vi "build-diode-scan-pts - v3.vi"(4 "Bar In PD Angle":dbl=180.5 format="%#_13g", 5 "Test Start Delay (s)":dbl=60.0, 6 "Bar In Brewster Angle":dbl=45.0 format="%#_13g", 7 "queue in":T2(array[cluster]), 8 "PD Y":cluster{"stop":dbl, "start":dbl, "step":dbl}, 9 "PD X":cluster{"stop":dbl, "start":dbl, "step":dbl}, 10 "Bar Y":cluster{"stop":dbl, "start":dbl, "step":dbl}, 11 "Bar X":cluster{"stop":dbl, "start":dbl, "step":dbl}) -> (3 "queue out":T2(array[cluster]))   [LabVIEW 2024]
panel:
  in  "next-state-cluster":T1={"next-state"="", "mode-select"=enum."IR", "bypass-confirm"=FALSE, "PDX"=300.0, "PDY"=150.0, "BarX"=300.0, "BarY"=150.0, "BMA"=45.0, "PDA"=85.0, "bar-note"=FALSE}
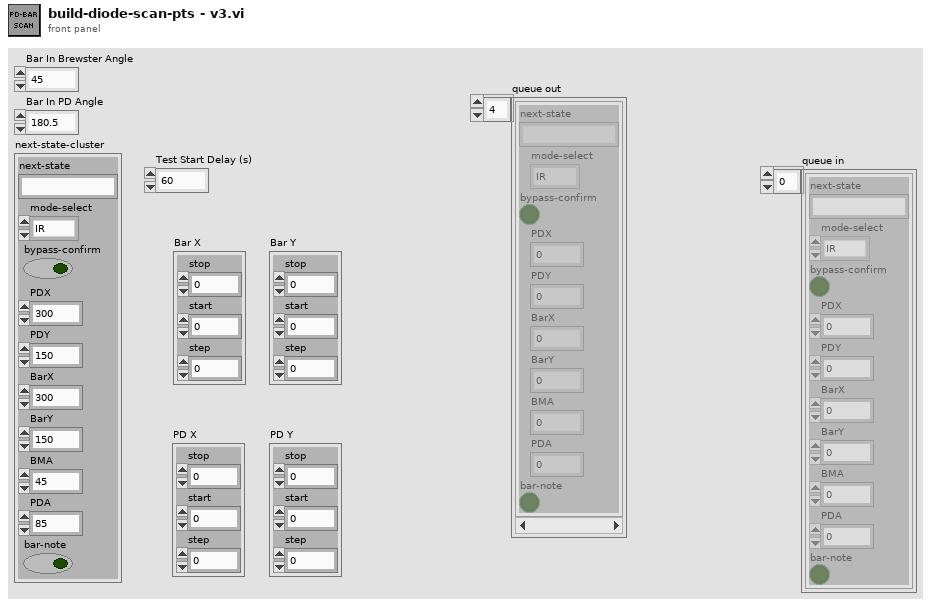
[diagram p1: front panel]
types:
  T1 = cluster{"next-state":string, "mode-select":enum32{"IR", "Pure", "Bulk", "Bar Out", "stored-loc", "custom"}, "bypass-confirm":bool, "PDX":dbl, "PDY":dbl, "BarX":dbl, "BarY":dbl, "BMA":dbl, "PDA":dbl, "bar-note":bool}
  T2 = cluster{"next-state":string, "mode-select":enum32{"IR", "Pure", "Bulk", "Bar Out", "stored-loc", "custom"}, "bypass-confirm":bool, "PDX":dbl, "PDY":dbl, "BarX":dbl, "BarY":dbl, "BMA":dbl, "PDA":dbl, "bar-note":bool}[]
  T3 = enum32{"IR", "Pure", "Bulk", "Bar Out", "stored-loc", "custom"}
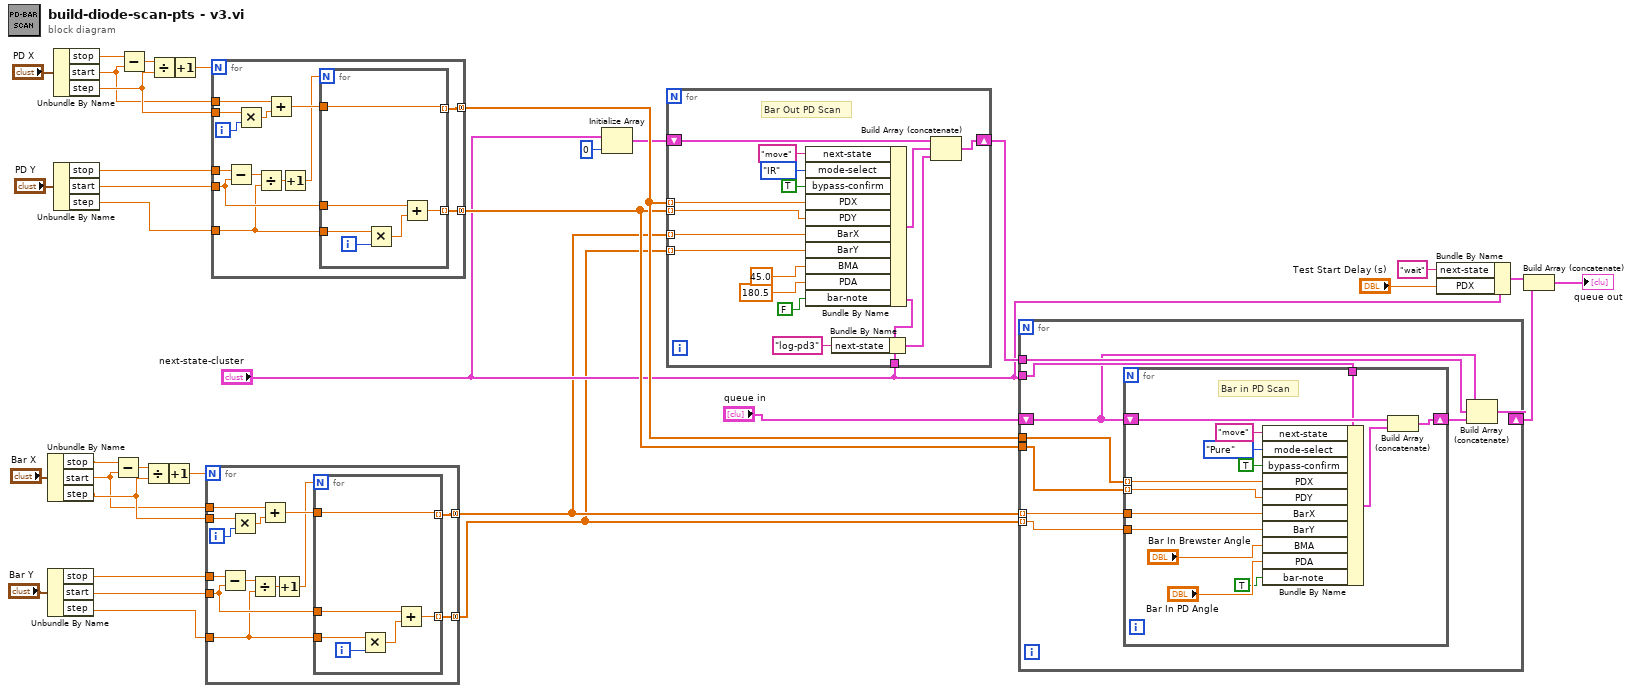
[diagram p0: block diagram]
diagram:
  n1 = Unbundle By Name("Bar X") -> ("stop"=w24:dbl, "start"=w25:dbl, "step"=w26:dbl)
  n2 = Unbundle By Name("Bar Y") -> ("stop"=w27:dbl, "start"=w28:dbl, "step"=w29:dbl)
  n3 = Unbundle By Name("PD X") -> ("stop"=w18:dbl, "start"=w19:dbl, "step"=w20:dbl)
  n4 = Unbundle By Name("PD Y") -> ("stop"=w21:dbl, "start"=w22:dbl, "step"=w23:dbl)
  n5 = Subtract(x=w24, y=w25) -> (x-y=w17:dbl)
  n6 = Subtract(x=w18, y=w19) -> (x-y=w12:dbl)
  n7 = Divide(x=w17, y=w26) -> (x/y=w16:dbl)
  n8 = Divide(x=w12, y=w20) -> (x/y=w13:dbl)
  n9 = Increment(x=w16) -> (x+1=w15:dbl)
  n10 = Increment(x=w13) -> (x+1=w14:dbl)
  n11 = for {
    N: w15 -> [_]
    tunnel: w25 -> [w48]
    tunnel: [w45] -> w2 mode=concatenating
    tunnel: [w44] -> w1 mode=concatenating
    tunnel: w26 -> [w40]
    tunnel: w27 -> [w39]
    tunnel: w28 -> [w38]
    tunnel: w29 -> [w37]
    i -> [w49]
    n12 = Subtract(x=w39, y=w38) -> (x-y=w43:dbl)
    n13 = Multiply(x=w40, y=w49) -> (x*y=w47:dbl)
    n14 = Divide(x=w43, y=w37) -> (x/y=w42:dbl)
    n15 = Add(x=w48, y=w47) -> (x+y=w46:dbl)
    n16 = Increment(x=w42) -> (x+1=w41:dbl)
    n17 = for {
      N: w41 -> [_]
      tunnel: w46 -> [w55]
      tunnel: [w55] -> w45 mode=indexing
      tunnel: [w52] -> w44 mode=indexing
      tunnel: w38 -> [w51]
      tunnel: w37 -> [w50]
      i -> [w53]
      n18 = Multiply(x=w50, y=w53) -> (x*y=w54:dbl)
      n19 = Add(x=w51, y=w54) -> (x+y=w52:dbl)
    }
  }
  n20 = for {
    N: w14 -> [_]
    tunnel: w19 -> [w67]
    tunnel: [w64] -> w9 mode=concatenating
    tunnel: [w63] -> w8 mode=concatenating
    tunnel: w20 -> [w59]
    tunnel: w21 -> [w58]
    tunnel: w22 -> [w57]
    tunnel: w23 -> [w56]
    i -> [w68]
    n21 = Subtract(x=w58, y=w57) -> (x-y=w62:dbl)
    n22 = Multiply(x=w59, y=w68) -> (x*y=w66:dbl)
    n23 = Divide(x=w62, y=w56) -> (x/y=w61:dbl)
    n24 = Add(x=w67, y=w66) -> (x+y=w65:dbl)
    n25 = Increment(x=w61) -> (x+1=w60:dbl)
    n26 = for {
      N: w60 -> [_]
      tunnel: w65 -> [w74]
      tunnel: [w74] -> w64 mode=indexing
      tunnel: [w71] -> w63 mode=indexing
      tunnel: w57 -> [w70]
      tunnel: w56 -> [w69]
      i -> [w72]
      n27 = Multiply(x=w69, y=w72) -> (x*y=w73:dbl)
      n28 = Add(x=w70, y=w73) -> (x+y=w71:dbl)
    }
  }
  n29 = Initialize Array("next-state-cluster", 0 ("dimension size")) -> (w6:T2)
  n30 = for {
    tunnel: w9 -> [w90] mode=indexing
    tunnel: w8 -> [w89] mode=indexing
    shift-right: [w82] -> w11
    shift-left: w6 -> [w84]
    tunnel: "next-state-cluster" -> [w78]
    tunnel: w2 -> [w76] mode=indexing
    tunnel: w1 -> [w75] mode=indexing
    # "Bar Out PD Scan"
    n31 = Bundle By Name(cluster=w78, "next-state"="move", "mode-select"=T3."IR", "bypass-confirm"=TRUE, "PDX"=w90, "PDY"=w89, "BarX"=w76, "BarY"=w75, "BMA"=45.0, "PDA"=180.5, "bar-note"=FALSE) -> (w83:T1)
    n32 = Bundle By Name(cluster=w78, "next-state"="log-pd3") -> (w79:T1)
    n33 = Build Array (concatenate)(w84, w83, w79) -> (w82:T2)
  }
  n34 = for {
    tunnel: w2 -> [w99] mode=indexing
    tunnel: w1 -> [w98] mode=indexing
    shift-right: [w96] -> w10
    shift-left: "queue in" -> [w91]
    tunnel: w11 -> [w95]
    tunnel: w9 -> [w94]
    tunnel: w8 -> [w93]
    tunnel: "next-state-cluster" -> [w92]
    n35 = for {
      tunnel: w94 -> [w113] mode=indexing
      tunnel: w93 -> [w112] mode=indexing
      shift-right: [w106] -> w97
      shift-left: w91 -> [w108]
      tunnel: w99 -> [w103]
      tunnel: w98 -> [w102]
      tunnel: w92 -> [w101]
      # "Bar in PD Scan"
      n36 = Bundle By Name(cluster=w101, "next-state"="move", "mode-select"=T3."Pure", "bypass-confirm"=TRUE, "PDX"=w113, "PDY"=w112, "BarX"=w103, "BarY"=w102, "BMA"="Bar In Brewster Angle", "PDA"="Bar In PD Angle", "bar-note"=TRUE) -> (w107:T1)
      n37 = Build Array (concatenate)(w108, w107) -> (w106:T2)
    }
    n38 = Build Array (concatenate)(w91, w95, w97) -> (w96:T2)
  }
  n39 = Bundle By Name(cluster="next-state-cluster", "next-state"="wait", "PDX"="Test Start Delay (s)") -> (w34:T1)
  n40 = Build Array (concatenate)(w34, w10) -> (→"queue out":T2)
